vi "Stop Sub Loop.vi"(8 "error in (no error)":errorcluster, 11 "Measurement in":refnum<class "Measurement.lvclass">) -> (0 "error out":errorcluster, 2 "Stop?":bool, 3 "Measurement out":refnum<class "Measurement.lvclass">)   [LabVIEW 2016, in "Measurement Actor.lvlib" / "Measurement.lvclass"]
uses:
  Measurement.lvclass
  Measurement.lvclass/Measurement.ctl
panel:
  in  "Wait":i32
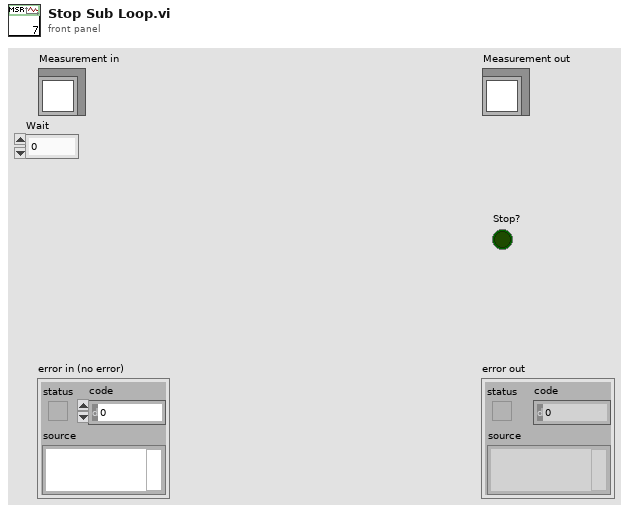
[diagram p1: front panel]
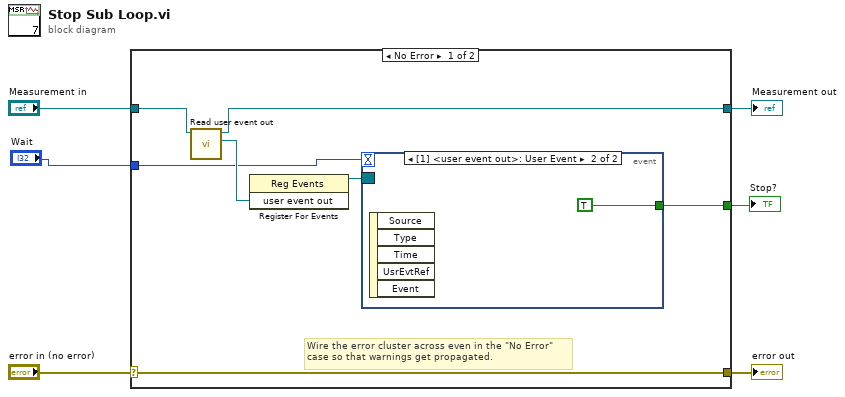
[diagram p0: block diagram]
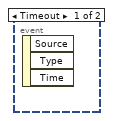
[diagram p2: hidden frame]
diagram:
  n1 = case shown="No Error" "error in (no error)" {
    selector: "error in (no error)" -> [w13 w16]
    tunnel: [w13 w16] -> w5
    tunnel: [w11 w15] -> w3
    tunnel: "Measurement in" -> [w12 w15]
    tunnel: "Wait" -> [w8 _]
    tunnel: [w7 _] -> w1
    frame No Error {
      # "Wire the error cluster across even in the \"No Error\"\ncase so that warnings get propagated."
      n2 = call "Read user event out.vi"("Measurement in"=w12) -> ("user event out"=w10:refnum<user-event>, "Measurement out"=w11:refnum<class "Measurement.lvclass">)  [unwired: 8 in, 1 out]
      n3 = register-events(w10) -> (reference out=w9:refnum<event-registration>)  [unwired: 2 in, 1 out]
      n4 = event shown="[1] <user event out>: User Event" {
        selector: w9 -> [_ _]
        dyn-events: _ -> [_ _]
        timeout: w8 -> [_ _]
        tunnel: [_ TRUE ("Stop?")] -> w7
        event Timeout {
          n5 = event-data() -> ()  [unwired: 1 in, 3 out]
        }
        event User Event {
          n6 = event-data() -> ()  [unwired: 1 in, 5 out]
        }
      }
    }
    frame Error {
    }
  }
  "error out" <- w5
  "Measurement out" <- w3
  "Stop?" <- w1
